vi "MotorMove.vi"(3 "Motor":string="PI1-SHUTTER", 4 "Movement":i32, 9 "error in (no error)":errorcluster) -> (0 "Motor out":string="PI1-SHUTTER", 6 "error out":errorcluster)   [LabVIEW 2009]
uses:
  Controls/MotorCommand.ctl
  Controls/MotorCommandBasic.ctl
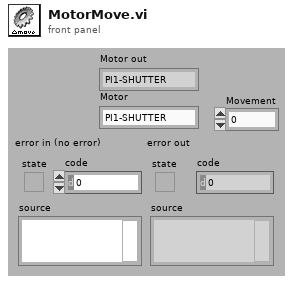
[diagram p1: front panel]
types:
  T1 = typedef "MotorCommandBasic.ctl" = enum16{"SELECT", "MOVE", "PREMOVE", "TURBO", "POS", "NAMED", "INIT", "STOP", "OFF", "SPEED", "QUIT"}
  T2 = typedef "MotorCommand.ctl" = cluster{"Motor":string, "Command":T1, "Movement":i32, "Name":string, "Param":cluster{"VMIN":i32, "VMAX":i32, "ACC":i32}, "Ok?":refnum<k4>, "Go!":refnum<k4>}
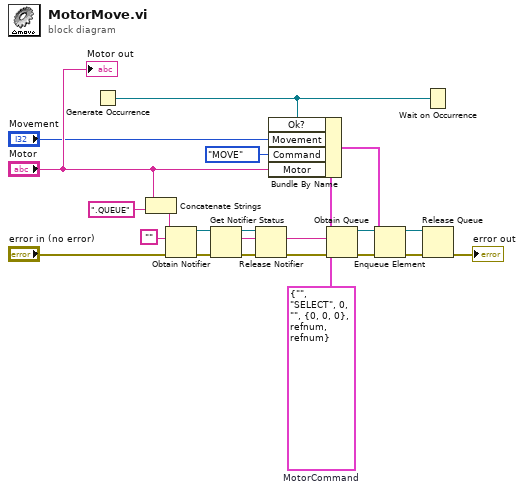
[diagram p0: block diagram]
diagram:
  w19 = T2 {"Motor"="", "Command"=enum."SELECT", "Movement"=0, "Name"="", "Param"={"VMIN"=0, "VMAX"=0, "ACC"=0}, "Ok?"=refnum, "Go!"=refnum}  # MotorCommand
  n1 = Generate Occurrence() -> (w1:refnum<k4>)
  n2 = Concatenate Strings("Motor", ".QUEUE") -> (w10:string)
  n3 = Obtain Notifier(name (unnamed)=w10, notification data type="", error in (no error)="error in (no error)") -> (notifier out=w11:refnum<notifier>, error out=w12:errorcluster)  [unwired: 1 in, 1 out]
  n4 = Get Notifier Status(notifier=w11, error in (no error)=w12) -> (notifier out=w14:refnum<notifier>, current notification=w7:string, error out=w15:errorcluster)  [unwired: 2 out]
  n5 = Release Notifier(notifier=w14, error in (no error)=w15) -> (error out=w8:errorcluster)  [unwired: 3 out]
  n6 = Bundle By Name(cluster=w19, "Ok?"=w1, "Movement"="Movement", "Command"=MotorCommandBasic."MOVE", "Motor"="Motor") -> (w18:T2)
  n7 = Obtain Queue(name (unnamed)=w7, element data type=w19, error in (no error)=w8) -> (queue out=w21:refnum<queue>, error out=w20:errorcluster)  [unwired: 2 in, 1 out]
  n8 = Enqueue Element(queue=w21, element=w18, error in (no error)=w20) -> (queue out=w16:refnum<queue>, error out=w17:errorcluster)  [unwired: 2 out]
  n9 = Wait on Occurrence(2:w1) -> ()  [unwired: 3 out]
  n10 = Release Queue(queue=w16, error in (no error)=w17) -> (error out=→"error out":errorcluster)  [unwired: 3 out]
  "Motor out" <- "Motor"
